vi "increment error.vi"(8 "error in (no error)":errorcluster, 11 "SP in":refnum<class "Save messages PGserver.lvclass">) -> (0 "error out":errorcluster, 2 "N errors":i32, 3 "SP out":refnum<class "Save messages PGserver.lvclass">)   [LabVIEW 2019, in "Save messages PGserver.lvclass"]
uses:
  Save messages PGserver.lvclass
  Save messages PGserver.lvclass/Save messages PGserver.ctl
  Modbus/Eth Status/Eth Status.lvlib
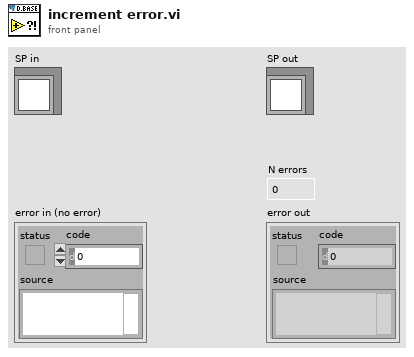
[diagram p1: front panel]
types:
  T1 = typedef "Eth Status.lvlib/Status.ctl" = cluster{"Set_state_com":refnum<data-value>, "start":refnum<data-value>, "WrEn":refnum<data-value>, "errors":refnum<data-value>, "connect":refnum<data-value>, "state":refnum<data-value>}
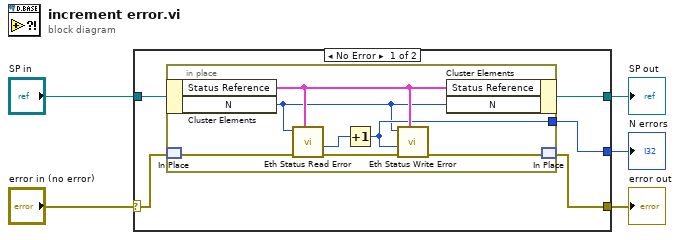
[diagram p0: block diagram]
diagram:
  n1 = case shown="No Error" "error in (no error)" {
    selector: "error in (no error)" -> [w9 w18]
    tunnel: [w8 w18] -> w4
    tunnel: [w6 w19] -> w1
    tunnel: "SP in" -> [w10 w19]
    tunnel: [w7 _] -> w3
    frame No Error {
      n2 = in-place {
        in-place-border: [w13] -> w7
        n3 = in-place-cluster #1(w10) -> ("Status Reference"=w16:T1, "N"=w11:i32)
        n4 = in-place-match #2(w9) -> (w17:errorcluster)
        n5 = call "Eth Status Read Error.vi"("Status Reference"=w16, "error in (no error)"=w17, "N"=w11) -> ("error out"=w15:errorcluster, "Error"=w14:i32)  [unwired: 7 in]
        n6 = Increment(x=w14) -> (x+1=w13:i32)
        n7 = call "Eth Status Write Error.vi"("Status Reference"=w16, "error in (no error)"=w15, "Errors"=w13, "N"=w11) -> ("error out"=w12:errorcluster)  [unwired: 7 in]
        n8 = in-place-cluster #1("Status Reference"=w16, "N"=w11) -> (w6:refnum<class "Save messages PGserver.lvclass">)
        n9 = in-place-match #2(w12) -> (w8:errorcluster)
      }
    }
    frame Error {
    }
  }
  "error out" <- w4
  "N errors" <- w3
  "SP out" <- w1
